vi "IRkHzInit131202_SD.vi"() -> ()   [LabVIEW 2015]
panel:
  in  "Dat in 10ns":u32=1
  # "Valeur pour la photodiode: 93970\n\nValeur pour l'absorption transitoire Elyse: 1"
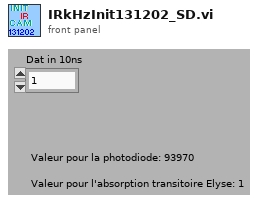
[diagram p1: front panel]
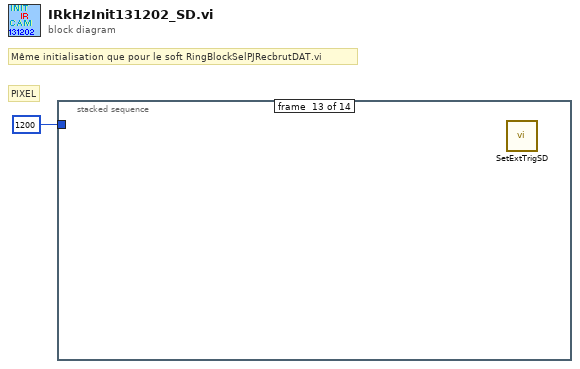
[diagram p0: block diagram]
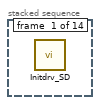
[diagram p2: hidden frame]
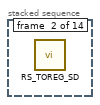
[diagram p3: hidden frame]
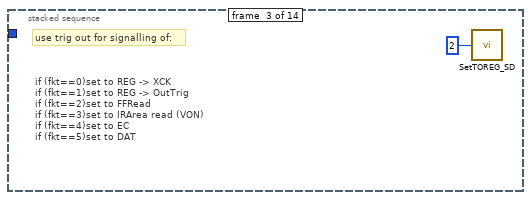
[diagram p4: hidden frame]
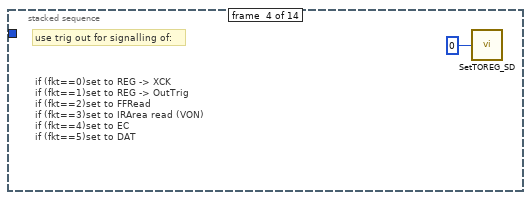
[diagram p5: hidden frame]
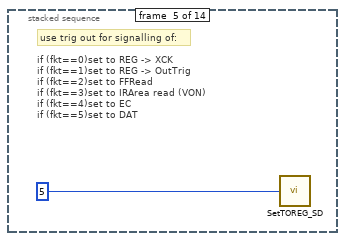
[diagram p6: hidden frame]
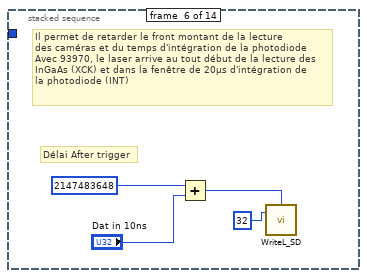
[diagram p7: hidden frame]
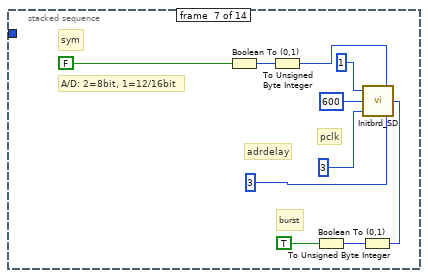
[diagram p8: hidden frame]
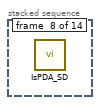
[diagram p9: hidden frame]
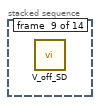
[diagram p10: hidden frame]
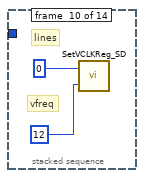
[diagram p11: hidden frame]
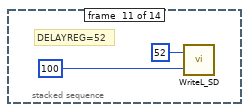
[diagram p12: hidden frame]
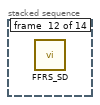
[diagram p13: hidden frame]
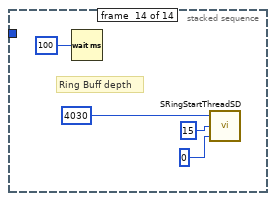
[diagram p14: hidden frame]
diagram:
  # "Même initialisation que pour le soft RingBlockSelPJRecbrutDAT.vi"
  # "PIXEL"
  n1 = stacked-sequence {
    tunnel: u32 1200 -> [_ _ _ _ _ _ _ _ _ _ _ _ _ _]
    frame #0 {
      n2 = call "Initdrv_SD.vi"() -> ()  [unwired: 1 in]
    }
    frame #1 {
      n3 = call "RS_TOREG_SD.vi"() -> ()  [unwired: 1 in]
    }
    frame #2 {
      # "use trig out for signalling of:"
      # "if (fkt==0)set to REG -> XCK\nif (fkt==1)set to REG -> OutTrig\nif (fkt==2)set to FFRead\nif (fkt==3)set to IRArea read (VON)\nif (fkt==4)set to EC\nif (fkt==5)set to DAT"
      n4 = call "SetTOREG_SD.vi"("fkt"=u8 2) -> ()
    }
    frame #3 {
      # "use trig out for signalling of:"
      # "if (fkt==0)set to REG -> XCK\nif (fkt==1)set to REG -> OutTrig\nif (fkt==2)set to FFRead\nif (fkt==3)set to IRArea read (VON)\nif (fkt==4)set to EC\nif (fkt==5)set to DAT"
      n5 = call "SetTOREG_SD.vi"("fkt"=u8 0) -> ()
    }
    frame #4 {
      # "use trig out for signalling of:"
      # "if (fkt==0)set to REG -> XCK\nif (fkt==1)set to REG -> OutTrig\nif (fkt==2)set to FFRead\nif (fkt==3)set to IRArea read (VON)\nif (fkt==4)set to EC\nif (fkt==5)set to DAT"
      n6 = call "SetTOREG_SD.vi"("fkt"=u8 5) -> ()
    }
    frame #5 {
      # "Il permet de retarder le front montant de la lecture \ndes caméras et du temps d'intégration de la photodiode\nAvec 93970, le laser arrive au tout début de la lecture des\nInGaAs (XCK) et dans la fenêtre de 20µs d'intégration de \nla photodiode (INT)"
      # "Délai After trigger"
      n7 = Add(x=u32 2147483648 ("offset"), y="Dat in 10ns") -> (x+y=w7:u32)
      n8 = call "WriteL_SD.vi"("val"=w7, "offset"=u32 32) -> ()
    }
    frame #6 {
      # "adrdelay"
      # "pclk"
      # "A/D: 2=8bit, 1=12/16bit"
      # "burst"
      # "sym"
      n9 = Boolean To (0,1)(Boolean=FALSE) -> (0, 1=w12:i16)
      n10 = To Unsigned Byte Integer(number=w12) -> (unsigned 8bit integer=w13:u8)
      n11 = Boolean To (0,1)(Boolean=TRUE) -> (0, 1=w11:i16)
      n12 = To Unsigned Byte Integer(number=w11) -> (unsigned 8bit integer=w10:u8)
      n13 = call "Initbrd_SD.vi"("AdrDelay"=u32 3, "burst"=w10, "sym"=w13, "waits"=u32 3, "pixel"=u32 600, "flag816"=u32 1) -> ()
    }
    frame #7 {
      n14 = call "IsPDA_SD.vi"() -> ()  [unwired: 1 in]
    }
    frame #8 {
      n15 = call "V_off_SD.vi"() -> ()  [unwired: 1 in]
    }
    frame #9 {
      # "vfreq"
      # "lines"
      n16 = call "SetVCLKReg_SD.vi"("vfreq"=u8 12, "lines"=u32 0) -> ()
    }
    frame #10 {
      # "DELAYREG=52"
      n17 = call "WriteL_SD.vi"("val"=u32 100, "offset"=u32 52) -> ()
    }
    frame #11 {
      n18 = call "FFRS_SD.vi"() -> ()  [unwired: 1 in]
    }
    frame #12 {
      n19 = call "SetExtTrigSD.vi"() -> ()  [unwired: 1 in]
    }
    frame #13 {
      # "Ring Buff depth"
      n20 = Wait (ms)(milliseconds to wait=u32 100) -> ()  [unwired: 1 out]
      n21 = call "SRingStartThreadSD.vi"("releasems"=i16 0, "threadp"=u32 15, "ringdepth"=u32 4030) -> ()
    }
  }
